vi "Row Index to State String.vi"(8 "error in (no error)":errorcluster, 10 "Row Index":i32, 11 "StateMachine in":refnum<class "StateMachine.lvclass">) -> (0 "error out":errorcluster, 1 "Row Index found?":bool, 2 "State String":string)   [LabVIEW 2018, in "State Machine.lvlib" / "StateMachine.lvclass"]
uses:
  StateMachine.lvclass
  StateMachine.lvclass/StateMachine.ctl
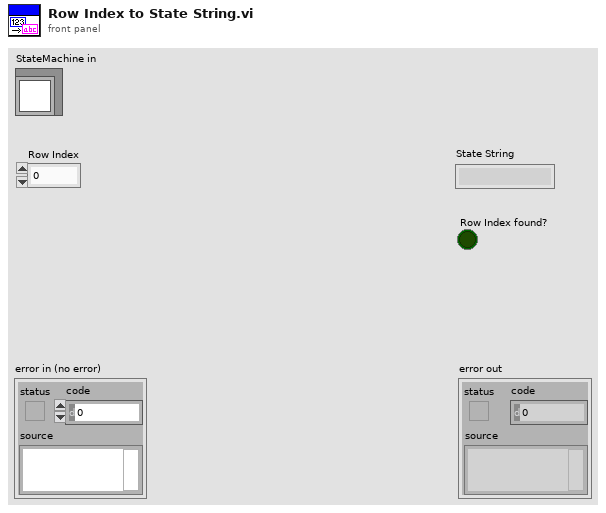
[diagram p1: front panel]
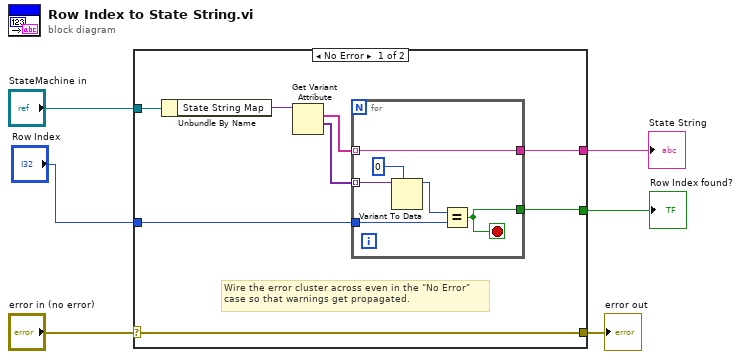
[diagram p0: block diagram]
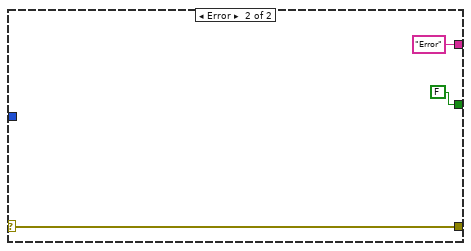
[diagram p2: hidden frame]
diagram:
  n1 = case shown="No Error" "error in (no error)" {
    selector: "error in (no error)" -> [w14 w23]
    tunnel: [w14 w23] -> w5
    tunnel: "StateMachine in" -> [w13 _]
    tunnel: "Row Index" -> [w9 _]
    tunnel: [w7 "Error"] -> w2
    tunnel: [w8 FALSE] -> w1
    frame No Error {
      # "Wire the error cluster across even in the \"No Error\"\ncase so that warnings get propagated."
      n2 = Unbundle By Name(w13) -> ("State String Map"=w12:variant)
      n3 = Get Variant Attribute(Variant=w12) -> (names=w11:string[], values=w10:variant[])  [unwired: 3 in, 2 out]
      n4 = for {
        tunnel: w11 -> [w15] mode=indexing
        tunnel: w10 -> [w19] mode=indexing
        tunnel: w9 -> [w17]
        tunnel: [w16] -> w8
        tunnel: [w15] -> w7
        stop <- w16 stop-if-true
        n5 = Variant To Data(type=0, Variant=w19) -> (data=w18:i32)  [unwired: 1 in, 1 out]
        n6 = Equal?(x=w18, y=w17) -> (x = y?=w16:bool)
      }
    }
    frame Error {
    }
  }
  "error out" <- w5
  "State String" <- w2
  "Row Index found?" <- w1
